vi "Read AMI.vi"() -> ()   [LabVIEW 2017]
uses:
  <instrlib>/Samwontech TEMP2xxx/Samwontech TEMP2xxx.lvlib
panel:
  out "Version-Revision":string
  out "Model Name":string
  out "Information":string
  in  "VISA resource name":refnum<visa-resource-name>
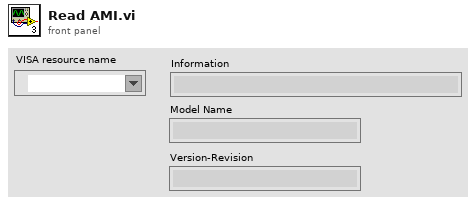
[diagram p1: front panel]
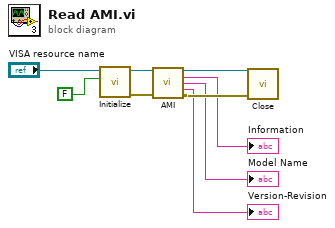
[diagram p0: block diagram]
diagram:
  n1 = call <instrlib>:"Initialize.vi"("ID Query (True)"=FALSE, "VISA resource name"="VISA resource name") -> ("error out"=w6:errorcluster, "VISA resource name out"=w7:refnum<visa-resource-name>)  [unwired: 8 in]
  n2 = call <instrlib>:"AMI.vi"("VISA resource name"=w7, "error in"=w6) -> ("VISA resource name out"=w5:refnum<visa-resource-name>, "Information"=→"Information":string, "Model Name"=→"Model Name":string, "Version-Revision"=→"Version-Revision":string, "error out"=w4:errorcluster)  [unwired: 9 in]
  n3 = call <instrlib>:"Close.vi"("error in (no error)"=w4, "VISA resource name"=w5) -> ()  [unwired: 9 in, 1 out]
